vi "depth_servo_ui.vi"() -> ()   [LabVIEW 2013]
panel:
  in  "Integral gain":sgl=0.02 min=0 max=0.1 step=0.001 format="%#_3p"
  in  "Max offset":sgl=1500.0 format="%#_3p"
  in  "Depth servo mode":enum16{"Limit", "Servo", "Off"}(ring)
  in  "Depth goal":sgl(slide) min=0 max=5000 step=100 scale=0.0..1000.0
  # "These globals are used to connect depth_servo.vi in goal loop to the user interface."
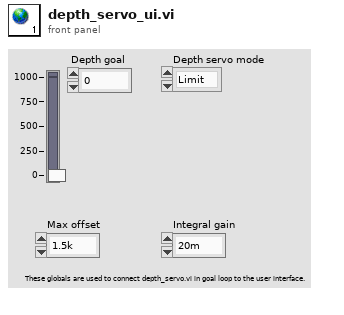
[diagram p1: front panel]
diagram:
